vi "Discovery Loop Async.vi"(11 "DiscoveryService in":refnum<class "NodeDiscovery.lvclass">) -> ()   [LabVIEW 2020, in "Vecto.lvlib" / "NodeDiscovery.lvclass"]
uses:
  NodeDiscovery.lvclass
  proto/Discovery/Class/Msg.lvclass
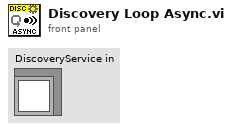
[diagram p1: front panel]
types:
  T1 = typedef "Service.lvlib/Data.ctl" = cluster{"type":T2, "port":i32}
  T2 = typedef "ServiceType.lvlib/Enumeration.ctl" = enum16{"SERVICETYPE_UNKNOWN", "SERVICETYPE_TCPSERVER", "SERVICETYPE_HTTPSERVER"}
  T3 = typedef "Discovery.lvlib/Data.ctl" = cluster{"node_id":u32, "name":string, "ip":u32, "status":string, "services":T1[], "system":string, "cluster":string}
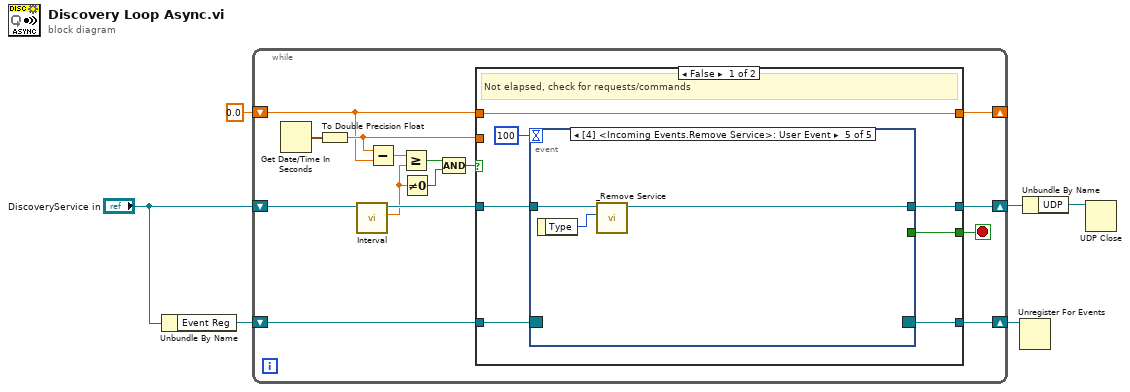
[diagram p0: block diagram]
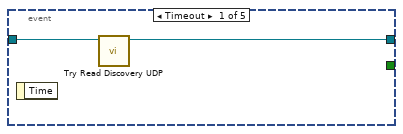
[diagram p2: hidden frame]
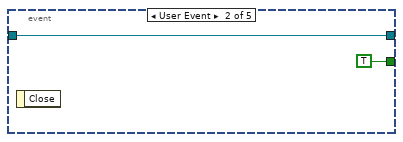
[diagram p3: hidden frame]
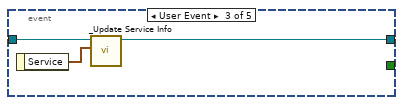
[diagram p4: hidden frame]
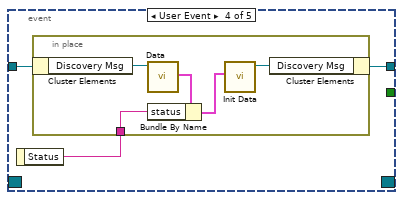
[diagram p5: hidden frame]
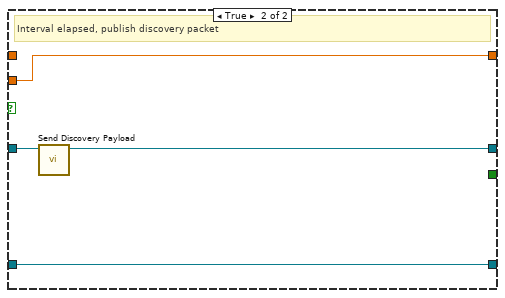
[diagram p6: hidden frame]
diagram:
  n1 = Unbundle By Name("DiscoveryService in") -> ("Event Reg"=w4:refnum<event-registration>)
  n2 = while {
    shift-right: [w15] -> _
    shift-left: 0.0 -> [w17]
    shift-right: [w14] -> w2
    shift-left: "DiscoveryService in" -> [w19]
    shift-right: [w12] -> w3
    shift-left: w4 -> [w13]
    stop <- w11 stop-if-true
    n3 = Get Date/Time In Seconds() -> (seconds since 1Jan1904=w21:timestamp)
    n4 = To Double Precision Float(number=w21) -> (double precision float=w18:dbl)
    n5 = call "Interval.vi"("DiscoveryService in"=w19) -> ("Interval S"=w8:dbl, "DiscoveryService out"=w10:refnum<class "NodeDiscovery.lvclass">)  [unwired: 8 in, 1 out]
    n6 = Subtract(x=w18, y=w17) -> (x-y=w20:dbl)
    n7 = Greater Or Equal?(x=w20, y=w8) -> (x >= y?=w16:bool)
    n8 = Not Equal To 0?(x=w8) -> (x != 0?=w7:bool)
    n9 = Compound Arithmetic op=AND(w16, w7) -> (w9:bool)
    n10 = case shown="False" w9 {
      tunnel: w10 -> [w26 w49]
      tunnel: w18 -> [_ w50]
      tunnel: w17 -> [w28 _]
      tunnel: [w28 w50] -> w15
      tunnel: [w25 w48] -> w14
      tunnel: w13 -> [w24 w47]
      tunnel: [w23 w47] -> w12
      tunnel: [w22 _] -> w11
      frame False {
        # "Not elapsed, check for requests/commands"
        n11 = event shown="[4] <Incoming Events.Remove Service>: User Event" {
          selector: w24 -> [_ _ _ _ _]
          dyn-events: [_ _ _ _ _] -> w23
          timeout: 100 -> [_ _ _ _ _]
          tunnel: w26 -> [w30 w32 w35 w38 w46]
          tunnel: [w29 w32 w33 w36 w44] -> w25
          tunnel: [_ TRUE _ _ _] -> w22
          event Timeout {
            n12 = event-data() -> ()  [unwired: 1 in, 1 out]
            n13 = call "Try Read Discovery UDP.vi"("DiscoveryService in"=w30) -> ("DiscoveryService out"=w29:refnum<class "NodeDiscovery.lvclass">)  [unwired: 9 in, 1 out]
          }
          event User Event {
            n14 = event-data() -> ()  [unwired: 1 in, 1 out]
          }
          event User Event {
            n15 = event-data() -> ("Service"=w34:T1)  [unwired: 1 in]
            n16 = call "_Update Service Info.vi"("Service"=w34, "DiscoveryService in"=w35) -> ("DiscoveryService out"=w33:refnum<class "NodeDiscovery.lvclass">)  [unwired: 8 in, 1 out]
          }
          event User Event {
            n17 = event-data() -> ("Status"=w37:string)  [unwired: 1 in]
            n18 = in-place {
              in-place-border: w37 -> [w41]
              n19 = in-place-cluster #1(w38) -> ("Discovery Msg"=w43:refnum<class "Msg.lvclass">)
              n20 = call "Data.vi"("PB Msg Template in"=w43) -> ("Data"=w42:T3)  [unwired: 8 in, 2 out]
              n21 = Bundle By Name(cluster=w42, "status"=w41) -> (w40:T3)
              n22 = call "Init Data.vi"("Data"=w40) -> ("Msg out"=w39:refnum<class "Msg.lvclass">)  [unwired: 10 in]
              n23 = in-place-cluster #1("Discovery Msg"=w39) -> (w36:refnum<class "NodeDiscovery.lvclass">)
            }
          }
          event User Event {
            n24 = event-data() -> ("Type"=w45:T2)  [unwired: 1 in]
            n25 = call "_Remove Service.vi"("Type"=w45, "DiscoveryService in"=w46) -> ("DiscoveryService out"=w44:refnum<class "NodeDiscovery.lvclass">)  [unwired: 8 in, 1 out]
          }
        }
      }
      frame True {
        # "Interval elapsed, publish discovery packet"
        n26 = call "Send Discovery Payload.vi"("DiscoveryService in"=w49) -> ("DiscoveryService out"=w48:refnum<class "NodeDiscovery.lvclass">)  [unwired: 9 in, 1 out]
      }
    }
  }
  n27 = Unregister For Events(event registration refnum=w3) -> ()  [unwired: 1 in, 1 out]
  n28 = Unbundle By Name(w2) -> ("UDP"=w1:refnum<k16>)
  n29 = UDP Close(connection ID=w1) -> ()  [unwired: 1 in, 2 out]
